vi "Save To File.vi"(7 "error in (no error)":errorcluster, 9 "File":path, 10 "ByRef Variant Repsitory in":refnum<data-value>) -> (0 "error out":errorcluster)   [LabVIEW 2015, in "ByRef Variant Repository.lvlib"]
uses:
  ByRef Variant Repository.lvlib
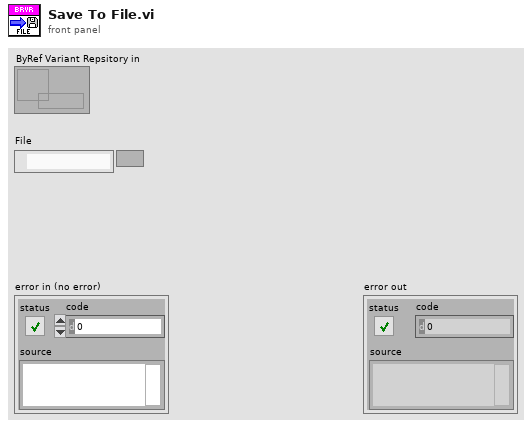
[diagram p1: front panel]
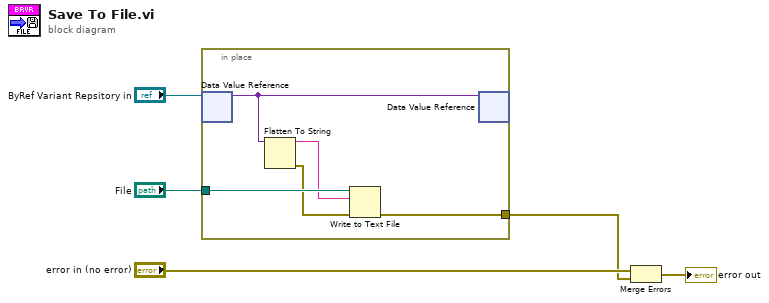
[diagram p0: block diagram]
diagram:
  n1 = in-place {
    in-place-border: "File" -> [w9]
    in-place-border: [w6] -> w1
    n2 = in-place-dvr #1("ByRef Variant Repsitory in") -> (w10:variant)  [unwired: 1 out]
    n3 = Flatten To String(anything=w10) -> (data string=w8:string, error out=w7:errorcluster)  [unwired: 3 in, 1 out]
    n4 = Write to Text File(file (use dialog)=w9, text=w8, error in=w7) -> (error out=w6:errorcluster)  [unwired: 1 in, 2 out]
    n5 = in-place-dvr #1(w10) -> ()  [unwired: 2 out]
  }
  n6 = Merge Errors("error in (no error)", w1) -> (→"error out":errorcluster)
